vi "Volt Reader Trigger8.vi"() -> ()   [LabVIEW 2014]
uses:
  <vilib>/Utility/error.llb/DialogType.ctl
  <vilib>/_DAQmxBase/Internals/DAQmxBase Create Channel (AI-Voltage-Basic).vi
  <vilib>/_DAQmxBase/Internals/DAQmxBase Timing (Sample Clock).vi
  <vilib>/measure/mamon.llb/Trigger Detection for 1 Channel.vi
  <vilib>/_DAQmxBase/Internals/DAQmxBase Read (Analog 2D DBL NChan NSamp).vi
  <vilib>/measure/NI_MAPro.lvlib
panel:
  out "size of output array":i32
  out "Buffer Full?":bool
  out "trigger location":dbl format="%#_2g"
  out "Waveform Graph 2":waveform(dbl)(graph)
  out "Waveform Graph":waveform(dbl)(graph)
  in  "Buffer (Seconds)":dbl
  out "Threshold":dbl
  in  "units":i32(ring)=10348 items=["Volts"=10348, "From Custom Scale"=10065]
  in  "stop":bool
  in  "physical channels":tag
  in  "maximum value":dbl=5.0 format="%0.2f"
  in  "minimum value":dbl=-5.0 format="%0.2f"
  in  "rate":i32=1000 caption="Sample Rate"
  # "The inputs above MUST BE\nPreset before running"
  # "NOTE: Just change the Y axis value"
  # "Make Sure that Buffer does not equal 0"
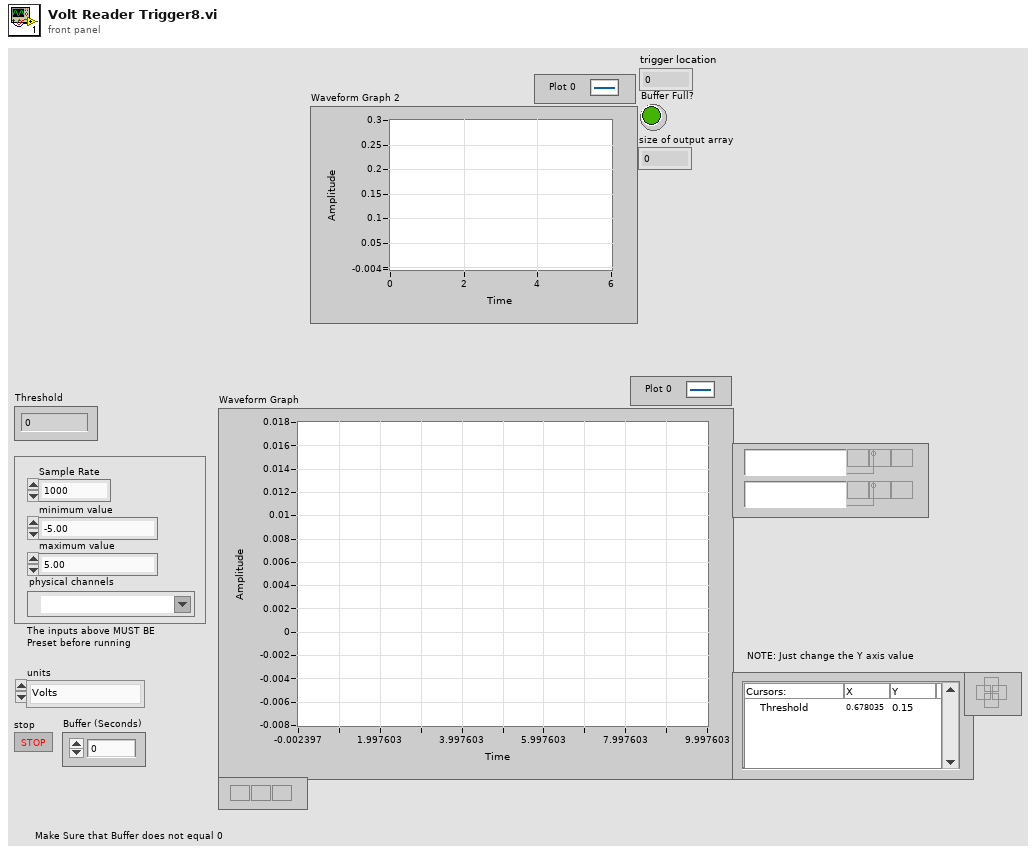
[diagram p1: front panel]
types:
  T1 = typedef "DialogType.ctl" = u16
  T2 = typedef "LVCursorListTypeDef.ctl" = cluster{"Name":string, "Color":u32, "Style":u8, "Point Style":u8, "Name Visible":bool, "Allow Drag":bool, "Cursor Mode":u32, "Plot":i32, "Index":i32, "Position":cluster{"X":dbl, "Y":dbl}, "X Scale":u32, "Y Scale":u32, "Watch Plots":i32[], "Watch All Plots":bool, "Plot Area":i32, "Label Offset":cluster{"X":dbl, "Y":dbl}}[]
  T3 = cluster{"Name":string, "Color":u32, "Style":u8, "Point Style":u8, "Name Visible":bool, "Allow Drag":bool, "Cursor Mode":u32, "Plot":i32, "Index":i32, "Position":cluster{"X":dbl, "Y":dbl}, "X Scale":u32, "Y Scale":u32, "Watch Plots":i32[], "Watch All Plots":bool, "Plot Area":i32, "Label Offset":cluster{"X":dbl, "Y":dbl}}
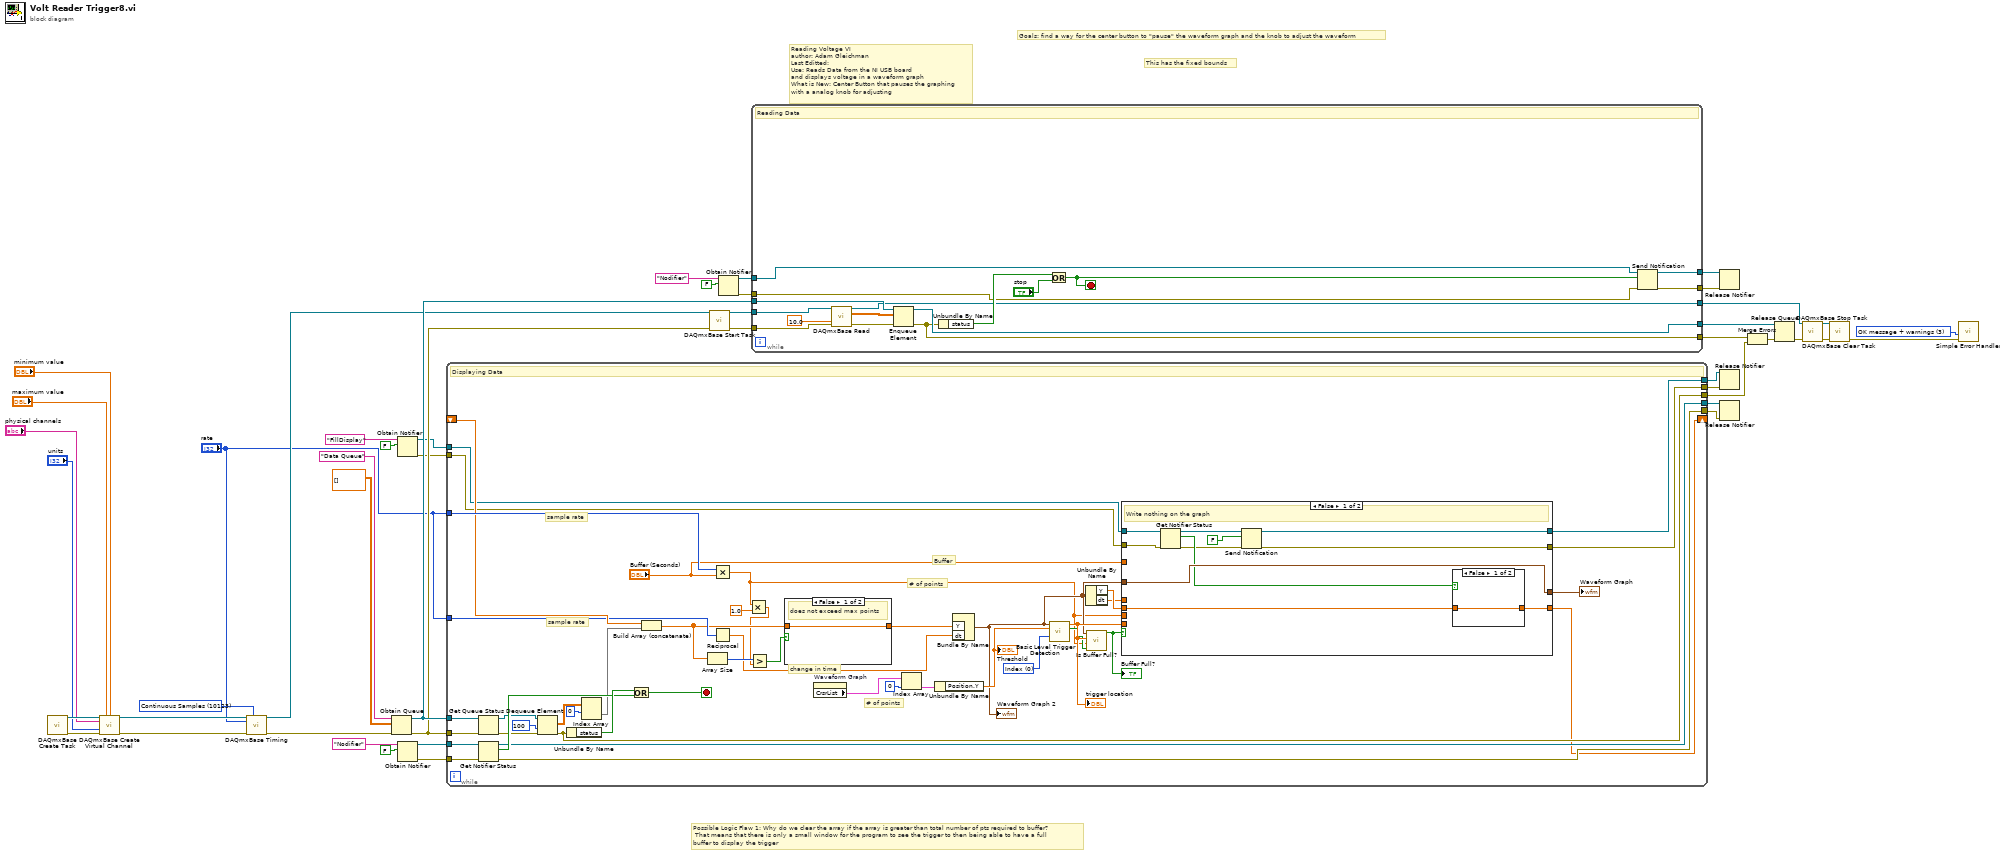
[diagram p0: block diagram]
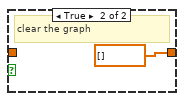
[diagram p2: hidden frame]
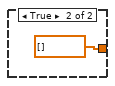
[diagram p3: hidden frame]
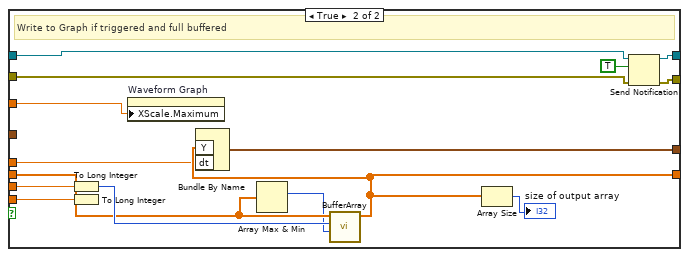
[diagram p4: hidden frame]
diagram:
  w23 = 10123 items=["Finite Samples"=10178, "Continuous Samples"=10123, "Hardware Timed Single Point"=12522] ("sample mode")
  w25 = T1 3 items=["no dialog", "OK message", "continue or stop message", "OK message + warnings", "continue/stop + warnings"] ("type of dialog (OK msg:1)")
  # "Possible Logic Flaw 1: Why do we clear the array if the array is greater than total number of pts required to buffer?\n That means that there is only a small window for the program to see the trigger to then being able to have a full\nbuffer to display the trigger"
  # "Goals: find a way for the center button to \"pause\" the waveform graph and the knob to adjust the waveform"
  # "This has the fixed bounds"
  # "Reading Voltage VI\nauthor: Adam Gleichman\nLast Editted: \nUse: Reads Data from the NI USB board\nand displays voltage in a waveform graph\nWhat is New: Center Button that pauses the graphing\nwith a analog knob for adjusting"
  n1 = call <vilib>:"DAQmxBase Create Task.vi"() -> ("task out"=w45:refnum<k21>, "error out"=w44:errorcluster)  [unwired: 5 in, 9 out]
  n2 = call-poly <vilib>:"DAQmxBase Create Virtual Channel.vi"("task in"=w45, "maximum value"="maximum value", "minimum value"="minimum value", "physical channels"="physical channels", "units"="units", "error in"=w44) -> ("task out"=w42:refnum<k21>, "error out"=w43:errorcluster)  [unwired: 3 in, 5 out]
  n3 = call-poly <vilib>:"DAQmxBase Timing.vi"("task/channels in"=w42, "sample mode"=w23, "rate"="rate", "error in"=w43) -> ("task out"=w11:refnum<k21>, "error out"=w10:errorcluster)  [unwired: 3 in, 7 out]
  n4 = Obtain Queue(name (unnamed)="Data Queue", element data type=dbl[][] [] ("data"), error in (no error)=w10) -> (queue out=w32:refnum<queue>, error out=w31:errorcluster)  [unwired: 2 in, 1 out]
  n5 = Obtain Notifier(name (unnamed)="FillDisplay", notification data type=FALSE) -> (notifier out=w6:refnum<notifier>, error out=w5:errorcluster)  [unwired: 2 in, 1 out]
  n6 = Obtain Notifier(name (unnamed)="Nodifier", notification data type=FALSE) -> (notifier out=w16:refnum<notifier>, error out=w14:errorcluster)  [unwired: 2 in, 1 out]
  n7 = while {
    tunnel: w32 -> [w91]
    tunnel: w31 -> [w80]
    tunnel: [w89] -> w30
    tunnel: w16 -> [w86]
    tunnel: w14 -> [w85]
    tunnel: [w83] -> w12
    tunnel: [w82] -> w13
    tunnel: "rate" -> [w63]
    tunnel: "rate" -> [w73]
    shift-right: [w71] -> _
    shift-left: _ -> [w70]
    tunnel: w6 -> [w60]
    tunnel: w5 -> [w59]
    tunnel: [w58] -> w2
    tunnel: [w57] -> w1
    stop <- w87 stop-if-true
    w68 = u16 0 items=["Index", "Time"] ("location mode")
    # "Buffer"
    # "change in time"
    # "# of points"
    # "# of points"
    # "sample rate"
    # "sample rate"
    # "Displaying Data"
    n8 = Get Queue Status(queue=w91, error in (no error)=w80) -> (queue out=w81:refnum<queue>, error out=w79:errorcluster)  [unwired: 1 in, 6 out]
    n9 = Get Notifier Status(notifier=w86, error in (no error)=w85) -> (notifier out=w83:refnum<notifier>, current notification=w84:bool, error out=w82:errorcluster)  [unwired: 2 out]
    n10 = Dequeue Element(queue=w81, timeout in ms (-1)=100, error in (no error)=w79) -> (element=w77:dbl[][], error out=w89:errorcluster)  [unwired: 2 out]
    n11 = Unbundle By Name(w89) -> ("status"=w88:bool)
    n12 = Index Array(array=w77, index (row)=0 ("index")) -> (element=w72:dbl[])  [unwired: 1 in]
    n13 = Or(x=w88, y=w84) -> (x .or. y?=w87:bool)
    n14 = Build Array (concatenate)(w70, w72) -> (w53:dbl[])
    n15 = Array Size(array=w53) -> (size(s)=w56:i32)
    n16 = Multiply(x=w73, y="Buffer (Seconds)") -> (x*y=w48:dbl)
    n17 = Reciprocal(x=w63) -> (1/x=w52:dbl)
    n18 = Multiply(x=w48, y=1.0) -> (x*y=w49:dbl)
    n19 = Greater?(x=w56, y=w49) -> (0:w55:bool)
    n20 = case shown="False" w55 {
      tunnel: [w92 dbl[] []] -> w54
      tunnel: w53 -> [w92 _]
      frame False {
        # "does not exceed max points"
      }
      frame True {
        # "clear the graph"
      }
    }
    n21 = property on="Waveform Graph" class="WFGraph (strict)"() -> ("CrsrList"=w75:T2)  [unwired: 2 in, 2 out]
    n22 = Index Array(array=w75, index=0) -> (element=w74:T3)
    n23 = Unbundle By Name(w74) -> ("Position.Y"=w69:dbl)
    "Threshold" <- w69
    n24 = Bundle By Name("Y"=w54, "dt"=w52) -> (w61:waveform(dbl))  [unwired: 1 in]
    "Waveform Graph 2" <- w61
    n25 = call-poly <vilib>:"Basic Level Trigger Detection.vi"("signal in"=w61, "level"=w69, "location mode"=w68) -> ("trigger location"=w66:dbl, "trigger detected?"=w51:bool)  [unwired: 10 in, 1 out]
    "trigger location" <- w66
    n26 = Unbundle By Name(w61) -> ("Y"=w65:dbl[], "dt"=w64:dbl)
    n27 = call "Is Buffer Full?.vi"("Triggered?"=w51, "Buffer in Points"=w48, "Index location"=w66, "output waveform"=w61) -> ("Buffer Full?"=w67:bool)  [unwired: 7 in]
    "Buffer Full?" <- w67
    n28 = case shown="False" w67 {
      tunnel: w48 -> [_ w121]
      tunnel: [w102 w113] -> w71
      tunnel: w66 -> [_ w119]
      tunnel: w65 -> [w103 w109]
      tunnel: w64 -> [_ w110]
      tunnel: [w104 w117] -> w62
      tunnel: w61 -> [w104 _]
      tunnel: w60 -> [w100 w116]
      tunnel: w59 -> [w101 w115]
      tunnel: [w95 w112] -> w58
      tunnel: [w94 w111] -> w57
      tunnel: "Buffer (Seconds)" -> [_ w107]
      frame False {
        # "Write nothing on the graph"
        n29 = Get Notifier Status(notifier=w100, error in (no error)=w101) -> (notifier out=w98:refnum<notifier>, current notification=w99:bool, error out=w97:errorcluster)  [unwired: 2 out]
        n30 = Send Notification(notification=FALSE, notifier=w98, error in (no error)=w97) -> (notifier out=w95:refnum<notifier>, error out=w94:errorcluster)
        n31 = case shown="False" w99 {
          tunnel: w103 -> [w105 _]
          tunnel: [w105 dbl[] []] -> w102
          frame False {
          }
          frame True {
          }
        }
      }
      frame True {
        # "Write to Graph if triggered and full buffered"
        n32 = To Long Integer(number=w121) -> (32bit integer=w120:i32)
        n33 = To Long Integer(number=w119) -> ()  [unwired: 1 out]
        n34 = property on="Waveform Graph" class="WFGraph (strict)"("XScale.Maximum"=w107) -> ()  [unwired: 2 in, 2 out]
        n35 = Array Max & Min(array=w109) -> (max index (indices)=w108:i32)  [unwired: 3 out]
        n36 = call "BufferArray.vi"("Index"=w108, "Total amount of Pts"=w120, "Input Y-values"=w109) -> ("Output Array"=w113:dbl[])  [unwired: 8 in]
        n37 = Bundle By Name("Y"=w113, "dt"=w110) -> (w117:waveform(dbl))  [unwired: 1 in]
        n38 = Array Size(array=w113) -> (size(s)=→"size of output array":i32)
        n39 = Send Notification(notification=TRUE, notifier=w116, error in (no error)=w115) -> (notifier out=w112:refnum<notifier>, error out=w111:errorcluster)
      }
    }
    "Waveform Graph" <- w62
  }
  n40 = call <vilib>:"DAQmxBase Start Task.vi"("task/channels in"=w11, "error in"=w31) -> ("task out"=w40:refnum<k21>, "error out"=w41:errorcluster)  [unwired: 12 out]
  n41 = Obtain Notifier(name (unnamed)="Nodifier", notification data type=FALSE) -> (notifier out=w19:refnum<notifier>, error out=w18:errorcluster)  [unwired: 2 in, 1 out]
  n42 = while "Data Reading Loop" {
    tunnel: w41 -> [w136]
    tunnel: w40 -> [w137]
    tunnel: w32 -> [w134]
    tunnel: [w131] -> w35
    tunnel: [w129] -> w34
    tunnel: [w127] -> w22
    tunnel: w19 -> [w125]
    tunnel: w18 -> [w124]
    tunnel: [w123] -> w8
    tunnel: [w122] -> w7
    stop <- w126 stop-if-true
    # "Reading Data"
    n43 = call-poly <vilib>:"DAQmxBase Read.vi"("task/channels in"=w137, "timeout"=10.0, "error in"=w136) -> ("task out"=w127:refnum<k21>, "data"=w132:dbl[][], "error out"=w135:errorcluster)  [unwired: 10 in]
    n44 = Enqueue Element(queue=w134, element=w132, error in (no error)=w135) -> (queue out=w131:refnum<queue>, error out=w129:errorcluster)  [unwired: 1 in, 1 out]
    n45 = Unbundle By Name(w129) -> ("status"=w128:bool)
    n46 = Or(x=w128, y="stop") -> (x .or. y?=w126:bool)
    n47 = Send Notification(notification=w126, notifier=w125, error in (no error)=w124) -> (notifier out=w123:refnum<notifier>, error out=w122:errorcluster)
  }
  n48 = Release Notifier(notifier=w8, error in (no error)=w7) -> ()  [unwired: 1 in, 3 out]
  n49 = Release Notifier(notifier=w2, error in (no error)=w1) -> ()  [unwired: 1 in, 3 out]
  n50 = Release Notifier(notifier=w12, error in (no error)=w13) -> ()  [unwired: 1 in, 3 out]
  n51 = Merge Errors(w34, w30) -> (w33:errorcluster)
  n52 = Release Queue(queue=w35, error in (no error)=w33) -> (error out=w29:errorcluster)  [unwired: 1 in, 2 out]
  n53 = call <vilib>:"DAQmxBase Stop Task.vi"("task/channels in"=w22, "error in"=w29) -> ("task out"=w28:refnum<k21>, "error out"=w27:errorcluster)  [unwired: 12 in]
  n54 = call <vilib>:"DAQmxBase Clear Task.vi"("task in"=w28, "error in"=w27) -> ("error out"=w26:errorcluster)  [unwired: 13 in]
  n55 = call <vilib>:"Simple Error Handler.vi"("type of dialog (OK msg:1)"=w25, "error in (no error)"=w26) -> ()  [unwired: 3 in, 5 out]
